vi "swerve_math.vi"(0 "Strafe":dbl(slide) scale=-1.0..1.0, 2 "Forwards":dbl(slide) scale=-1.0..1.0, 4 "Rotate":dbl(slide) scale=-1.0..1.0, 6 "Gyro":dbl) -> (20 "Drive FR":dbl, 21 "Azimuth FR":dbl, 22 "Drive FL":dbl, 23 "Azimuth FL":dbl, 24 "Drive BL":dbl, 25 "Azimuth BL":dbl, 26 "Drive BR":dbl, 27 "Azimuth BR":dbl)   [LabVIEW 2020]
uses:
  <vilib>/Analysis/coordinate.llb/Angle Units.ctl
  <vilib>/Analysis/coordinate.llb/2D Cartesian Coordinate Rotation (Scalar).vi
  <vilib>/Analysis/coordinate.llb/Wrap Angle (scalar).vi
  <vilib>/Analysis/NI_AALPro.lvlib
  <vilib>/Analysis/NI_AAL_Angle.lvlib
panel:
  out "Back Right":cluster{"X":dbl, "Y":dbl}[](graph)
  out "Back Left":cluster{"X":dbl, "Y":dbl}[](graph)
  out "Front Right":cluster{"X":dbl, "Y":dbl}[](graph)
  out "Front Left":cluster{"X":dbl, "Y":dbl}[](graph)
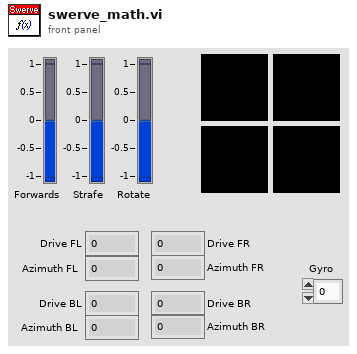
[diagram p1: front panel]
types:
  T1 = typedef "NI_AAL_Angle.lvlib/Angle Units.ctl" = i32
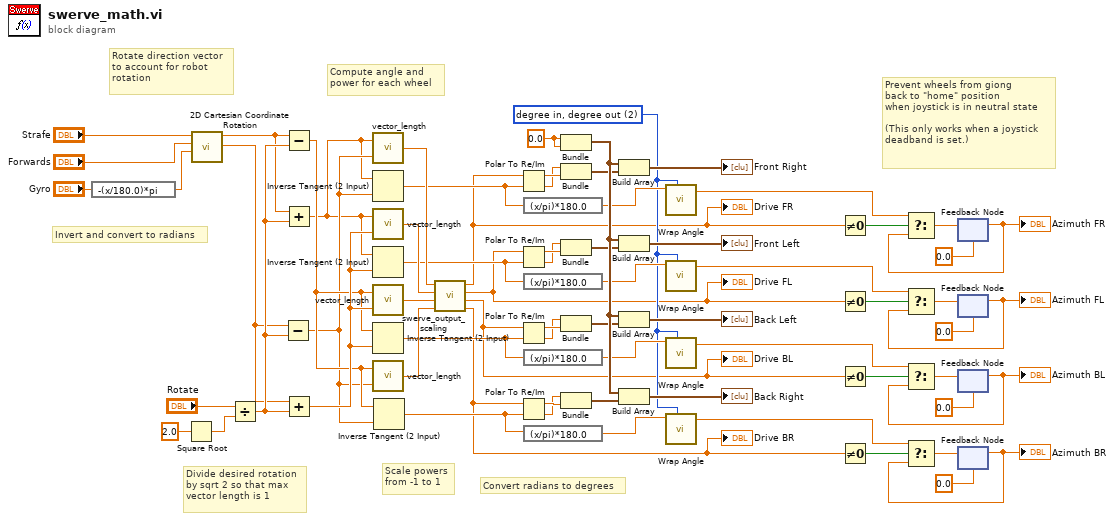
[diagram p0: block diagram]
diagram:
  w26 = T1 2 items=["radian in, radian out", "radian in, degree out", "degree in, degree out", "degree in, radian out"] ("angle units")
  w65 = 0.0 ("x")
  # "Prevent wheels from giong\nback to \"home\" position\nwhen joystick is in neutral state\n\n(This only works when a joystick\ndeadband is set.)"
  # "Divide desired rotation\nby sqrt 2 so that max\nvector length is 1"
  # "Convert radians to degrees"
  # "Scale powers\nfrom -1 to 1"
  # "Compute angle and \npower for each wheel"
  # "Rotate direction vector\nto account for robot \nrotation"
  # "Invert and convert to radians"
  n1 = expression code="-(x/180.0)*pi" ("degrees to radians")("Gyro") -> (w31:dbl)
  n2 = Square Root(x=2.0) -> (sqrt(x)=w69:dbl)
  n3 = call-poly <vilib>:"2D Cartesian Coordinate Rotation.vi"("theta"=w31, "y"="Forwards", "x"="Strafe") -> ("y out"=w33:dbl, "x out"=w34:dbl)  [unwired: 6 in, 1 out]
  n4 = Divide(x="Rotate", y=w69) -> (x/y=w66:dbl)
  n5 = Subtract(x=w33, y=w66) -> (x-y=w45:dbl)
  n6 = Subtract(x=w34, y=w66) -> (x-y=w46:dbl)
  n7 = Add(x=w34, y=w66) -> (x+y=w44:dbl)
  n8 = Add(x=w33, y=w66) -> (x+y=w47:dbl)
  n9 = call "vector_length.vi"("v_y"=w45, "v_x"=w44) -> ("||v||"=w55:dbl)
  n10 = Inverse Tangent (2 Input)(1:w45, 2:w44) -> (0:w48:dbl)
  n11 = call "vector_length.vi"("v_y"=w47, "v_x"=w44) -> ("||v||"=w54:dbl)
  n12 = Inverse Tangent (2 Input)(1:w47, 2:w44) -> (0:w49:dbl)
  n13 = call "vector_length.vi"("v_y"=w47, "v_x"=w46) -> ("||v||"=w53:dbl)
  n14 = Inverse Tangent (2 Input)(1:w47, 2:w46) -> (0:w50:dbl)
  n15 = call "vector_length.vi"("v_y"=w45, "v_x"=w46) -> ("||v||"=w52:dbl)
  n16 = Inverse Tangent (2 Input)(1:w45, 2:w46) -> (0:w51:dbl)
  n17 = call "swerve_output_scaling.vi"("d"=w52, "c"=w53, "b"=w54, "a"=w55) -> ("d scaled"=w5:dbl, "c scaled"=w4:dbl, "b scaled"=w3:dbl, "a scaled"=w2:dbl)  [unwired: 4 in]
  "Drive FR" <- w2
  "Drive FL" <- w3
  "Drive BL" <- w4
  "Drive BR" <- w5
  n18 = Polar To Re/Im(2:w48, 3:w2) -> (0:w42:dbl, 1:w43:dbl)
  n19 = Polar To Re/Im(2:w49, 3:w3) -> (0:w40:dbl, 1:w41:dbl)
  n20 = Polar To Re/Im(2:w50, 3:w4) -> (0:w38:dbl, 1:w39:dbl)
  n21 = Polar To Re/Im(2:w51, 3:w5) -> (0:w36:dbl, 1:w37:dbl)
  n22 = expression code="(x/pi)*180.0" ("radians to degrees")(w48) -> (w30:dbl)
  n23 = expression code="(x/pi)*180.0" ("radians to degrees")(w49) -> (w29:dbl)
  n24 = expression code="(x/pi)*180.0" ("radians to degrees")(w50) -> (w28:dbl)
  n25 = expression code="(x/pi)*180.0" ("radians to degrees")(w51) -> (w27:dbl)
  n26 = Bundle("x"=w65, "x"=w65) -> (w64:cluster{"x":dbl, "x":dbl})  [unwired: 1 in]
  n27 = Bundle(w42, w43) -> (w58:cluster{dbl, dbl})  [unwired: 1 in]
  n28 = Bundle(w40, w41) -> (w59:cluster{dbl, dbl})  [unwired: 1 in]
  n29 = Bundle(w38, w39) -> (w57:cluster{dbl, dbl})  [unwired: 1 in]
  n30 = Bundle(w36, w37) -> (w56:cluster{dbl, dbl})  [unwired: 1 in]
  n31 = Build Array(w64, w58) -> (→"Front Right":cluster{"x":dbl, "x":dbl}[])
  n32 = Build Array(w64, w59) -> (→"Front Left":cluster{"x":dbl, "x":dbl}[])
  n33 = Build Array(w64, w57) -> (→"Back Left":cluster{"x":dbl, "x":dbl}[])
  n34 = Build Array(w64, w56) -> (→"Back Right":cluster{"x":dbl, "x":dbl}[])
  n35 = call-poly <vilib>:"Wrap Angle.vi"("angle units"=w26, "angle in"=w30) -> ("angle out"=w24:dbl)  [unwired: 8 in, 1 out]
  n36 = call-poly <vilib>:"Wrap Angle.vi"("angle units"=w26, "angle in"=w29) -> ("angle out"=w15:dbl)  [unwired: 8 in, 1 out]
  n37 = call-poly <vilib>:"Wrap Angle.vi"("angle units"=w26, "angle in"=w28) -> ("angle out"=w14:dbl)  [unwired: 8 in, 1 out]
  n38 = call-poly <vilib>:"Wrap Angle.vi"("angle units"=w26, "angle in"=w27) -> ("angle out"=w13:dbl)  [unwired: 8 in, 1 out]
  n39 = Not Equal To 0?(x=w2) -> (x != 0?=w25:bool)
  n40 = Not Equal To 0?(x=w3) -> (x != 0?=w16:bool)
  n41 = Not Equal To 0?(x=w4) -> (x != 0?=w19:bool)
  n42 = Not Equal To 0?(x=w5) -> (x != 0?=w17:bool)
  n43 = feedback #1(0.0 ("angle out")) -> (w12:dbl)
  "Azimuth FR" <- w12
  n44 = Select(t=w24, s=w25, f=w12) -> (s? t:f=w23:dbl)
  n45 = feedback-in #1(w23) -> ()
  n46 = feedback #2(0.0 ("angle out")) -> (w11:dbl)
  "Azimuth FL" <- w11
  n47 = Select(t=w15, s=w16, f=w11) -> (s? t:f=w21:dbl)
  n48 = feedback-in #2(w21) -> ()
  n49 = feedback #3(0.0 ("angle out")) -> (w10:dbl)
  "Azimuth BL" <- w10
  n50 = Select(t=w14, s=w19, f=w10) -> (s? t:f=w20:dbl)
  n51 = feedback-in #3(w20) -> ()
  n52 = feedback #4(0.0 ("angle out")) -> (w9:dbl)
  "Azimuth BR" <- w9
  n53 = Select(t=w13, s=w17, f=w9) -> (s? t:f=w18:dbl)
  n54 = feedback-in #4(w18) -> ()
